vi "takeStep.vi"(7 "redTurn":i32, 8 "pos":i32[][](array[numeric]), 9 "exist":i32[][](array[numeric]), 10 "j":i32, 11 "i":i32) -> (1 "check":dbl, 2 "posNew":i32[][](array[numeric]), 3 "existNew":i32[][](array[numeric]))   [LabVIEW 2022 SP3, in "subvis.lvlib"]
uses:
  subvis.lvlib
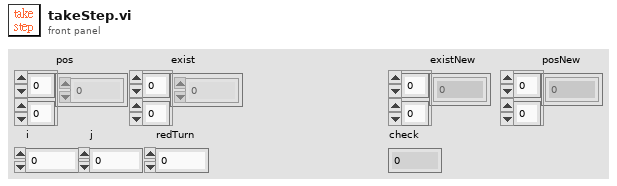
[diagram p1: front panel]
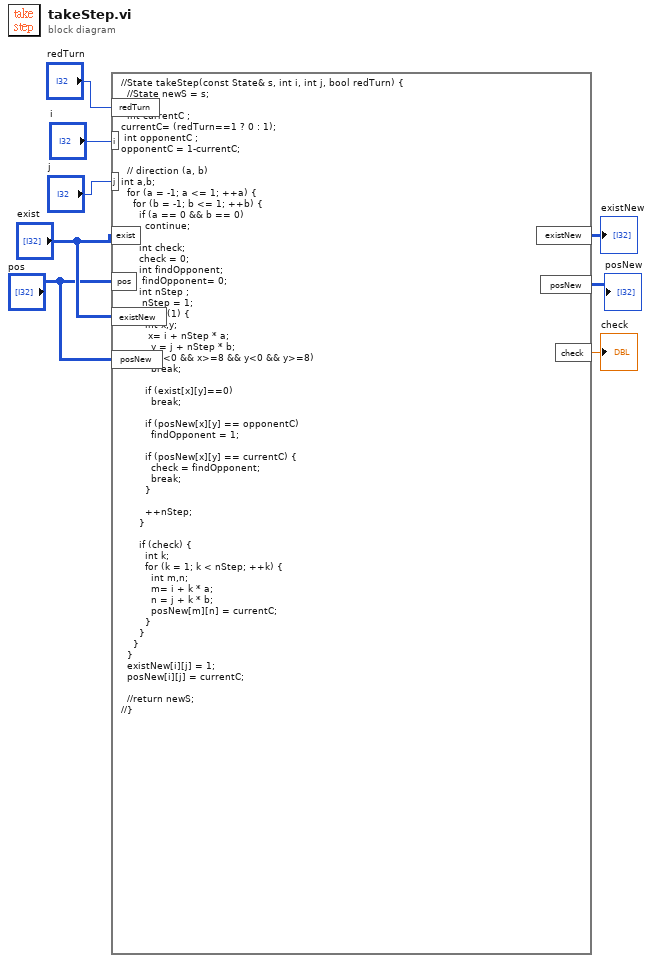
[diagram p0: block diagram]
diagram:
  n1 = formula code="//State takeStep(const State& s, int i, int j, bool redTurn) {\n  //State newS = s;\n\n  int currentC ;\ncurrentC= (redTurn==1 ? 0 : 1);\n int opponentC ;\nopponentC = 1-currentC;\n\n  // direction (a, b)\nint a,b;\n  for (a = -1; a <= 1; ++a) {\n    for (b = -1; b <= 1; ++b) {\n      if (a == 0 && b == 0)\n        continue;\n\n      int check;\n      check = 0;\n      int findOpponent; \n       findOpponent= 0;\n      int nStep ;\n       nStep = 1;\n      while (1) {\n        int x,y; \n         x= i + nStep * a;\n          y = j + nStep * b;\n        if (x<0 && x>=8 && y<0 && y>=8)\n          break;\n\n        if (exist[x][y]==0)\n          break;\n\n        if (posNew[x][y] == opponentC)\n          findOpponent = 1;\n\n        if (posNew[x][y] == currentC) {\n          check = findOpponent;\n          break;\n        }\n\n        ++nStep;\n      }\n\n      if (check) {\n        int k;\n        for (k = 1; k < nStep; ++k) {\n          int m,n;\n          m= i + k * a;\n          n = j + k * b;\n          posNew[m][n] = currentC;\n        }\n      }\n    }\n  }\n  existNew[i][j] = 1;\n  posNew[i][j] = currentC;\n\n  //return newS;\n//}"("pos"="pos", "exist"="exist", "redTurn"="redTurn", "i"="i", "j"="j", "existNew"="exist", "posNew"="pos") -> ("existNew"=→"existNew":i32[][], "posNew"=→"posNew":i32[][], "check"=→"check":dbl)
